vi "_emi_ SMLoop small droppin.vi"() -> ()   [LabVIEW 2010]
uses:
  Private/_emi_ SMLoop start condition.vi
  Private/_emi_ SMLoop Error Check.vi
  Basic/0 - General/Error/emi_Is Error.vi
  Error/emi_ Loop error state monitor.vi
  Private/_emi_SMLoop Register new.vi
  S&E reporting/emi_Send S&E Error message.vi
  Basic/0 - General/Error/emi_ Is Error state.vi
  emi_Read System ID.vi
  Loop control/Private/_emi_GFV Loop Linking.vi
  Loop control/Private/_emi_GFV Loop Enable.vi
  Private/_emi_ SMLoop Restart.vi
  Private/_emi_GFV App Close.vi
  Loop control/Private/_emi_GFV Loop Running.vi
  Private/_emi_GFV System ID.vi
  S&E reporting/Private/_emi_S&E Q Generator.vi
  <vilib>/Utility/error.llb/Clear Errors.vi
  Loop control/Private/_emi_GFV stop a loop so it can reset.vi
panel:
  in  "Loop ID":i32
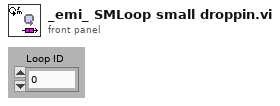
[diagram p1: front panel]
types:
  T1 = typedef "_emi_ SMLoop sates.ctl" = enum16{"Init", "Standby", "Start", "Normal Operation", "Stop", "Error Handling", "End", "Post"}
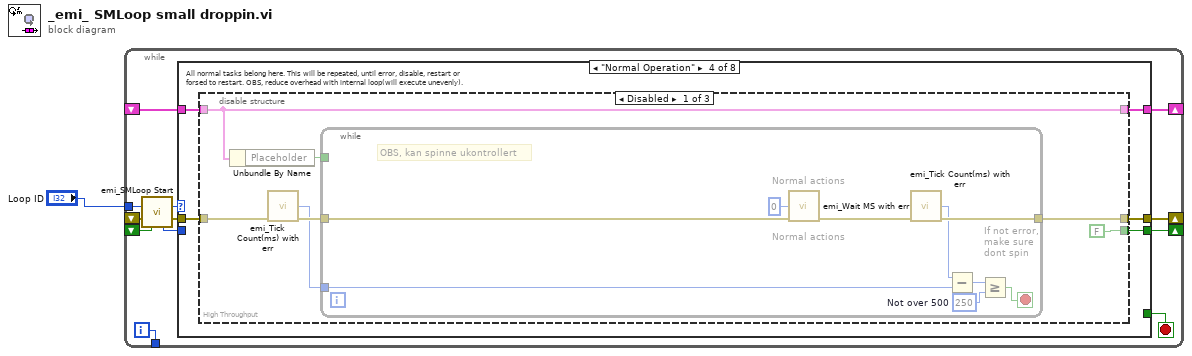
[diagram p0: block diagram]
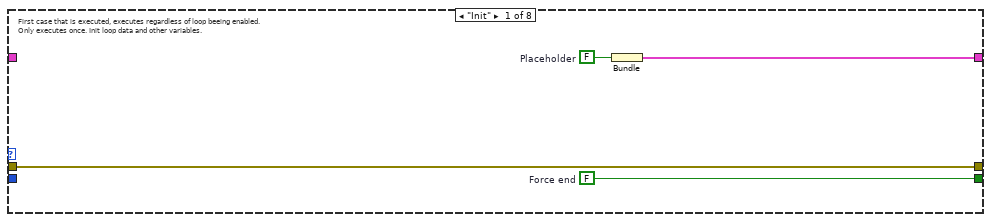
[diagram p2: hidden frame]
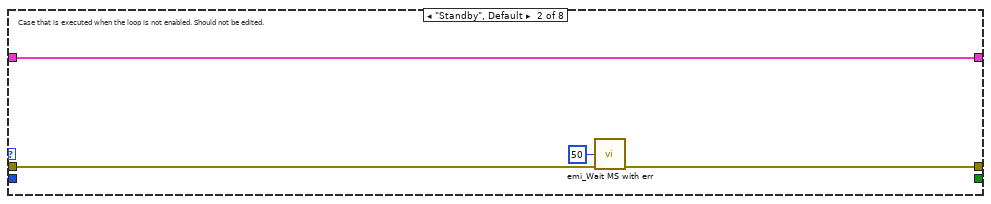
[diagram p3: hidden frame]
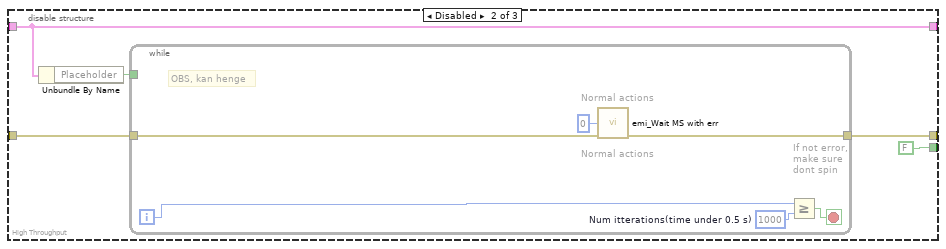
[diagram p5: hidden frame]
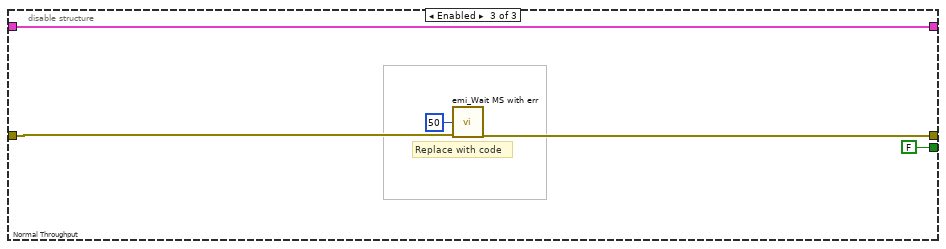
[diagram p6: hidden frame]
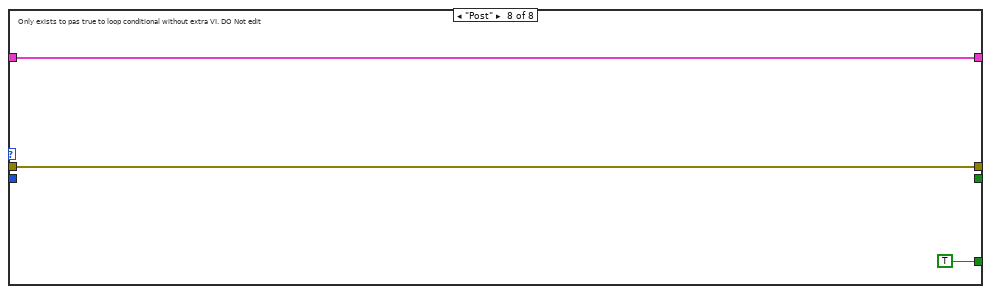
[diagram p10: hidden frame]
diagram:
  n1 = while {
    shift-right: [w13] -> _
    shift-left: _ -> [w9]
    shift-right: [w11] -> _
    shift-left: _ -> [w7]
    tunnel: [w10] -> _
    shift-right: [w8] -> _
    shift-left: _ -> [w3]
    tunnel: "Loop ID" -> [w4]
    i -> [w10]
    stop <- w12 stop-if-true
    n2 = call "emi_SMLoop Start.vi"("Loop ID"=w4, "error in (no error)"=w7, "Force Stop(F)"=w3) -> ("Loop command"=w5:T1, "error out"=w6:errorcluster, "Loop ID out"=w2:i32)  [unwired: 10 in]
    n3 = case shown="\"Normal Operation\"" w5 {
      tunnel: [w16 w18 w22 w26 w61 w64 w65 w68] -> w13
      tunnel: [_ _ _ _ _ _ _ TRUE] -> w12
      tunnel: w6 -> [w17 w20 w23 w28 w62 w63 w66 w69]
      tunnel: [w17 w19 w23 w27 w62 w63 w66 w69] -> w11
      tunnel: w9 -> [_ w18 w22 w25 w61 w64 w65 w68]
      tunnel: [w14 _ _ w24 _ _ _ _] -> w8
      tunnel: w2 -> [_ _ _ _ _ _ _ _]
      frame "Init" {
        w14 = FALSE  # Force end
        w15 = FALSE  # Placeholder
        # "First case that is executed, executes regardless of loop beeing enabled.\nOnly executes once. Init loop data and other variables."
        n4 = Bundle("Placeholder"=w15) -> (w16:cluster{"Placeholder":bool})  [unwired: 1 in]
      }
      frame "Standby", Default {
        # "Case that is executed when the loop is not enabled. Should not be edited."
        n5 = call "emi_Wait MS with err.vi"("milliseconds to wait(0)"=u32 50, "error in (no error)"=w20) -> ("error out"=w19:errorcluster)  [unwired: 13 in]
      }
      frame "Start" {
        # "Start or restart the loop. Should perform any init code. \nOpen channel and so on. Will perform each time the system is restarted."
      }
      frame "Normal Operation" {
        # "All normal tasks belong here. This will be repeated, until error, disable, restart or\nforsed to restart. OBS, reduce overhead with internal loop(will execute unevenly)."
        n6 = disable-structure shown="Disabled" {
          disable-tunnel: w28 -> [w32 w45 w58]
          disable-tunnel: [w34 w48 w57] -> w27
          disable-tunnel: [w35 w49 w60] -> w26
          disable-tunnel: w25 -> [w35 w49 w60]
          disable-tunnel: [FALSE ("Force End") FALSE ("Force End") FALSE ("Force End")] -> w24
          frame Disabled {
            # "High Throughput"
            n7 = Unbundle By Name(w35) -> ("Placeholder"=w33:bool)
            n8 = call "emi_Tick Count(ms) with err.vi"("error in (no error)"=w32) -> ("millisecond timer value"=w30:u32, "error out"=w31:errorcluster)  [unwired: 13 in]
            n9 = while {
              tunnel: w31 -> [w38]
              tunnel: [w44] -> w34
              tunnel: w33 -> [_]
              tunnel: w30 -> [w43]
              stop <- w37 stop-if-true
              w40 = u32 250  # Not over 500
              # "OBS, kan spinne ukontrollert"
              # "If not error,\nmake sure \ndont spin"
              # "Normal actions"
              # "Normal actions"
              n10 = call "emi_Wait MS with err.vi"("milliseconds to wait(0)"=u32 0, "error in (no error)"=w38) -> ("error out"=w39:errorcluster)  [unwired: 13 in]
              n11 = call "emi_Tick Count(ms) with err.vi"("error in (no error)"=w39) -> ("millisecond timer value"=w42:u32, "error out"=w44:errorcluster)  [unwired: 13 in]
              n12 = Subtract(x=w42, y=w43) -> (x-y=w41:u32)
              n13 = Greater Or Equal?(x=w41, y=w40) -> (x >= y?=w37:bool)
            }
          }
          frame Disabled {
            # "High Throughput"
            n14 = Unbundle By Name(w49) -> ("Placeholder"=w47:bool)
            n15 = while {
              tunnel: [w51] -> w48
              tunnel: w47 -> [_]
              tunnel: w45 -> [w52]
              i -> [w50]
              stop <- w54 stop-if-true
              w55 = u32 1000  # Num itterations(time under 0.5 s)
              # "OBS, kan henge"
              # "If not error,\nmake sure \ndont spin"
              # "Normal actions"
              # "Normal actions"
              n16 = call "emi_Wait MS with err.vi"("milliseconds to wait(0)"=u32 0, "error in (no error)"=w52) -> ("error out"=w51:errorcluster)  [unwired: 13 in]
              n17 = Greater Or Equal?(x=w50, y=w55) -> (x >= y?=w54:bool)
            }
          }
          frame Enabled {
            # "Replace with code"
            # "Normal Throughput"
            n18 = call "emi_Wait MS with err.vi"("milliseconds to wait(0)"=u32 50, "error in (no error)"=w58) -> ("error out"=w57:errorcluster)  [unwired: 13 in]
          }
        }
      }
      frame "Stop" {
        # "Stop the loop. May be restarted later. Close interfaces and the like"
      }
      frame "Error Handling" {
        # "Loop automaticaly returns here after error is found. If error is cleared, \nLoop wil continue as normal(if was operative when error."
      }
      frame "End" {
        # "Only executes at application end has. Should performa any action the loop \nneeds to finnish. Executes only once."
      }
      frame "Post" {
        # "Only exists to pas true to loop conditional without extra VI. DO Not edit"
      }
    }
  }
